vi "DualMotor.vi"() -> ()   [LabVIEW 2020]
uses:
  <vilib>/Platform/TimedLoop/XDataNode/timing_clust.ctl
  <vilib>/Platform/TimedLoop/XDataNode/nitl_modes.ctl
  <vilib>/Platform/TimedLoop/XDataNode/wakeup.ctl
  <vilib>/CANopenLib/CANOPEN.llb/CANopen Interface Create.vi
  <vilib>/CANopenLib/CANOPEN.llb/CANopen SDO Create.vi
  <vilib>/CANopenLib/CANOPEN.llb/CANopen SDO Write [I16].vi
  <vilib>/CANopenLib/CANOPEN.llb/CANopen SDO Close.vi
  <vilib>/CANopenLib/CANOPEN.llb/CANopen SYNC Create.vi
  <vilib>/CANopenLib/CANOPEN.llb/CANopen RPDO Create.vi
  <vilib>/CANopenLib/CANOPEN.llb/CANopen TPDO Create.vi
  <vilib>/CANopenLib/CANOPEN.llb/CANopen TPDO Start.vi
  <vilib>/CANopenLib/CANOPEN.llb/CANopen SYNC Start.vi
  <vilib>/CANopenLib/CANOPEN.llb/CANopen RPDO Start.vi
  <vilib>/imath/engines/lvmath/Functions/Error Handling/MergeErrorsWrapper.vi
  <vilib>/imath/engines/lvmath2/RunTimeEngine/NodeEndStatement/NIMS_NodeEndStatement_Output.vi
  <instcachedir>/0/NIMS_NodeEndStatement_Output_53EC0D466D134D7ABD903AC30B43404B.lvgen/NIMS_NodeEndStatement_Output_53EC0D466D134D7ABD903AC30B43404B_010.vi
  <vilib>/imath/engines/lvmath2/RunTimeEngine/ErrorHandling/NIMS_Finalize Error.vi
  <instcachedir>/0/NIMS_NodeEndStatement_Output_53EC0D466D134D7ABD903AC30B43404B.lvgen/NIMS_NodeEndStatement_Output_53EC0D466D134D7ABD903AC30B43404B_001.vi
  <vilib>/CANopenLib/CANOPEN.llb/CANopen Convert To Data [I16].vi
  <vilib>/CANopenLib/CANOPEN.llb/CANopen Fetch from Data [I16].vi
  <vilib>/CANopenLib/CANOPEN.llb/CANopen Fetch from Data [I32].vi
  <vilib>/CANopenLib/CANOPEN.llb/CANopen SYNC Close.vi
  <vilib>/CANopenLib/CANOPEN.llb/CANopen RPDO Close.vi
  <vilib>/CANopenLib/CANOPEN.llb/CANopen TPDO Close.vi
  <vilib>/CANopenLib/CANOPEN.llb/CANopen Interface Close.vi
  <vilib>/imath/engines/lvmath2/RunTimeEngine/BuiltInFunctions/mod/NIMS_mod_no_size_check.vi
  <instcachedir>/0/NIMS_mod_no_size_check_5393E3382FD241D281EEB71DA286C65B.lvgen/NIMS_mod_no_size_check_5393E3382FD241D281EEB71DA286C65B_001.vi
  <vilib>/FPGAPlugInAG/cRIO-9047/niLvFpga_Open_cRIO-9047.vi
  <vilib>/rvi/interface/common/dynamic/niFpgaDynamicAddResources.vi
  <vilib>/FPGAPlugInAG/Dynamic/niLvFpga_Download_Dynamic.vi
  <vilib>/FPGAPlugInAG/Dynamic/niLvFpga_Reset_Dynamic.vi
  <vilib>/FPGAPlugInAG/Dynamic/niLvFpga_Run_Dynamic.vi
  <vilib>/Utility/error.llb/Error Cluster From Error Code.vi
  <vilib>/rvi/errors/niLvFpgaAdjustHostInterfaceError.vi
  <vilib>/FPGAPlugInAG/Dynamic/niLvFpga_Close_Dynamic.vi
  <vilib>/Platform/TimedLoop/XDataNode/XDataNode.xnode
  <vilib>/rvi/interface/nirviOpenFPGA/nirviOpenFPGA.xnode
  PressureIO_12.vi
  <vilib>/rvi/interface/nirviMethod/nirviMethod.xnode
  <vilib>/rvi/interface/nirviReadWriteControl/nirviReadWriteControl.xnode
  <vilib>/rvi/interface/nirviCloseFPGA/nirviCloseFPGA.xnode
  <vilib>/Platform/TimedLoop/XDataNode/XDNodeRunTimeDep.lvlib
  NiFpgaLv.dll
  <vilib>/rvi/interface/Simulation/niFpgaSimulationCallBeginRW.vi
panel:
  out "L":dbl(graph)
  out "P2":dbl(graph)
  out "P1":dbl(graph)
  out "P2":dbl
  out "P1":dbl
  out "t":dbl
  out "Theta":dbl(graph)
  in  "自定义速度2":dbl
  in  "手动输入速度2":bool
  in  "自定义速度1":dbl
  in  "手动输入速度1":bool
  in  "SaveData?":bool=TRUE
  in  "文件路径（使用对话框）":path=path "C:/data.bin"
  in  "node-ID  2":u8=2 min=1 max=127 step=1
  out "completion code 5":u32
  in  "buffer size (0) 4":u16
  in  "TPDO channel 2":u8(ring)=2 items=["PDO 1", "PDO 2", "PDO 3", "PDO 4"]
  in  "Set Target Vilocity 2":i16
  in  "stop 2":bool
  out "timestamp 2":timestamp=timestamp(3824613290.037175 s since 1904-01-01)
  out "电机绝对位置 2":i32=443333152
  out "速度反馈值 2":i32=300
  in  "目标速度  2":i16
  out "转矩反馈值 0.1% 2":i16=40
  in  "buffer size (0) 3":u16=10
  in  "TPDO channel read 2":u8(ring)=1 items=["PDO 1", "PDO 2", "PDO 3", "PDO 4"]
  in  "RPDO channel write 2":u8(ring)=1 items=["PDO 1", "PDO 2", "PDO 3", "PDO 4"]
  in  "period (ms) 2":i64=10
  out "completion code 4":u32
  out "completion code 3":u32
  in  "batch SDO name 2":string="NiMotion_VM"
  out "completion code":u32
  in  "buffer size (0) 2":u16
  in  "TPDO channel":u8(ring)=2 items=["PDO 1", "PDO 2", "PDO 3", "PDO 4"]
  in  "Set Target Vilocity":i16
  in  "stop":bool
  out "timestamp":timestamp=timestamp(3833513217.6669617 s since 1904-01-01)
  out "电机绝对位置":i32=147770
  out "速度反馈值":i32
  in  "目标速度":i16
  out "转矩反馈值 0.1%":i16=10
  in  "buffer size (0)":u16=10
  in  "TPDO channel read":u8(ring)=1 items=["PDO 1", "PDO 2", "PDO 3", "PDO 4"]
  in  "RPDO channel write":u8(ring)=1 items=["PDO 1", "PDO 2", "PDO 3", "PDO 4"]
  in  "period (ms)":i64=10
  out "completion code 2":u32
  out "completion code 1":u32
  in  "batch SDO name":string="NiMotion_VM"
  in  "node-ID":u8=1 min=1 max=127 step=1
  in  "baud rate":u32(ring) items=["1 Mbit/s"=0, "800 kbit/s"=1, "500 kbit/s"=2, "250 kbit/s"=3, "125 kbit/s"=4, "50 kbit/s"=6, "20 kbit/s"=7, "10 kbit/s"=8]
  in  "CANopen interface":u32(ring) items=["CANopen01", "CANopen02", "CANopen03", "CANopen04", "CANopen05", "CANopen06", "CANopen07", "CANopen08", "CANopen09", "CANopen10", "CANopen11", "CANopen12", "CANopen13", "CANopen14", "CANopen15", "CANopen16", "CANopen17", "CANopen18", "CANopen19", "CANopen20", "CANopen21", "CANopen22", "CANopen23", "CANopen24", "CANopen25", "CANopen26", "CANopen27", "CANopen28", "CANopen29", "CANopen30", "CANopen31", "CANopen32"]
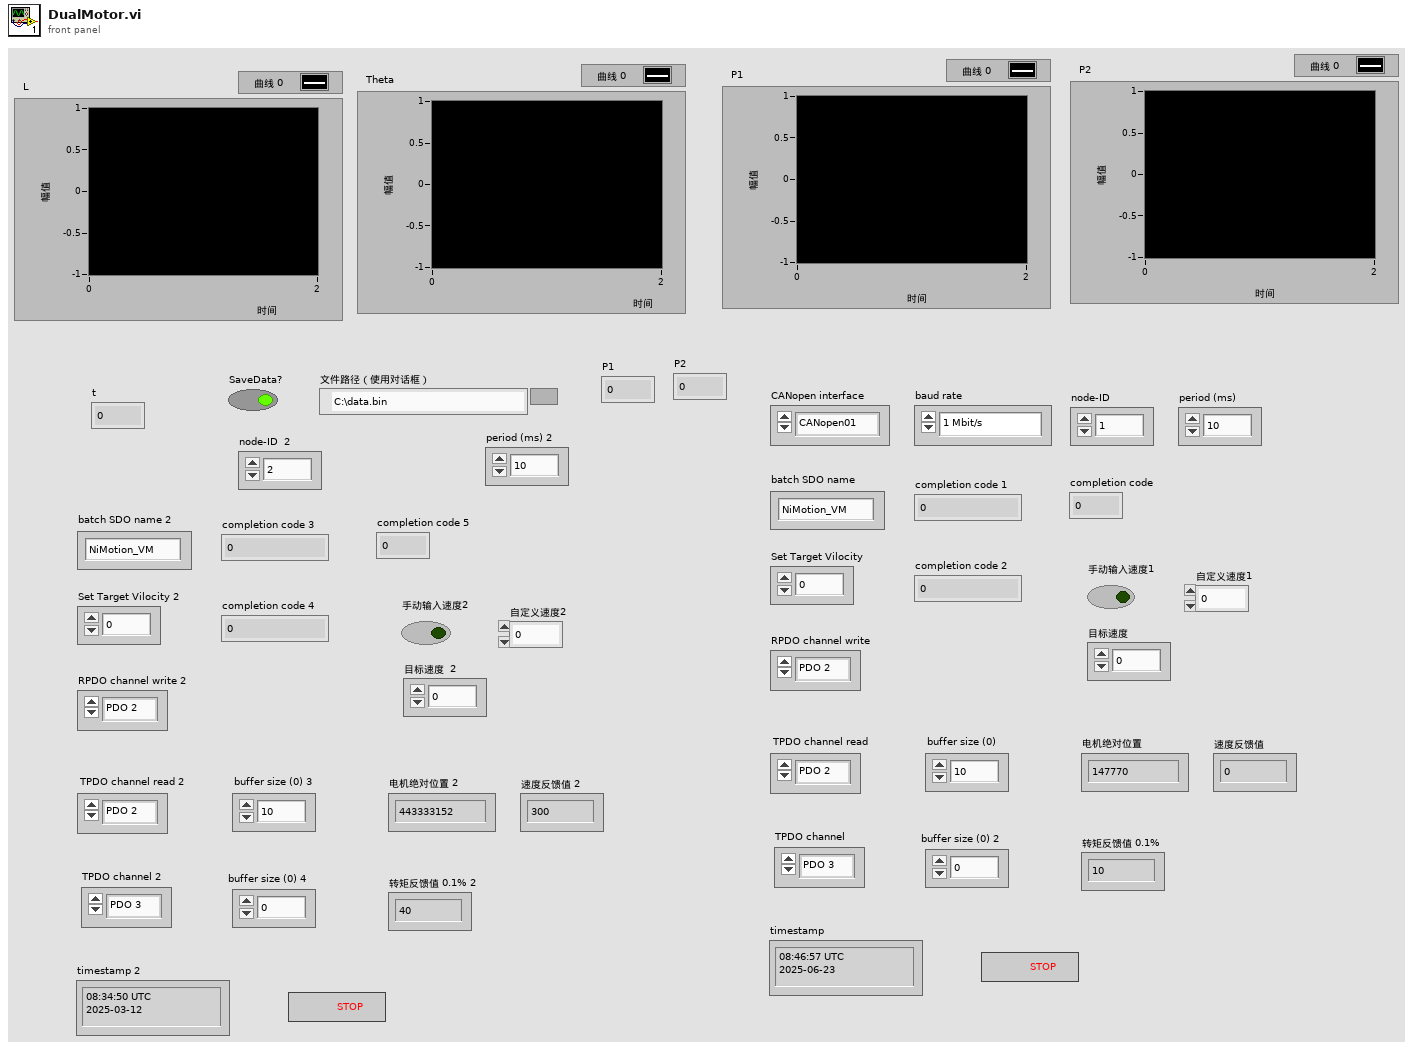
[diagram p1: front panel]
types:
  T1 = enum16{"open", "replace", "create", "open or create", "replace or create", "replace or create with confirmation"}
  T2 = enum16{"big-endian, network order", "native, host order", "little-endian"}
  T3 = typedef "XDNodeRunTimeDep.lvlib/timing_clust.ctl" = cluster{"Expected End [f-1]":u64, "Actual End [f-1]":u64, "Finished Late? [f-1]":bool, "Expected End [i-1]":u64, "Actual End [i-1]":u64, "Finished Late? [i-1]":bool, "Expected Start [i]":u64, "Actual Start [i]":u64, "Expected Start [f]":u64, "Actual Start [f]":u64, "Source Name":string, "Structure Name":string, "Period":i64, "Deadline":i64, "Offset":i64, "Start":i64, "Priority":i32, "Timeout":i32, "Mode":T4, "Wakeup Reason":T5, "Error":errorcluster, "Source Type":string, "Secondary Source Type":string, "Global End Time":u64, "Global Start Time":u64, "Frame Duration":u64, "Iteration Duration":u64, "Assigned CPU":i32, "I/O Scan Engine Mode":u32}
  T4 = typedef "XDNodeRunTimeDep.lvlib/nitl_modes.ctl" = enum32{"No Change", "Process missed periods, maintain original phase", "Discard missed periods, maintain original phase", "Process missed periods, ignore original phase", "Discard missed periods, ignore original phase"}
  T5 = typedef "XDNodeRunTimeDep.lvlib/wakeup.ctl" = enum32{"Normal", "Aborted", "Asynchronous wakeup", "Timing source error", "Timed loop error", "Timeout"}
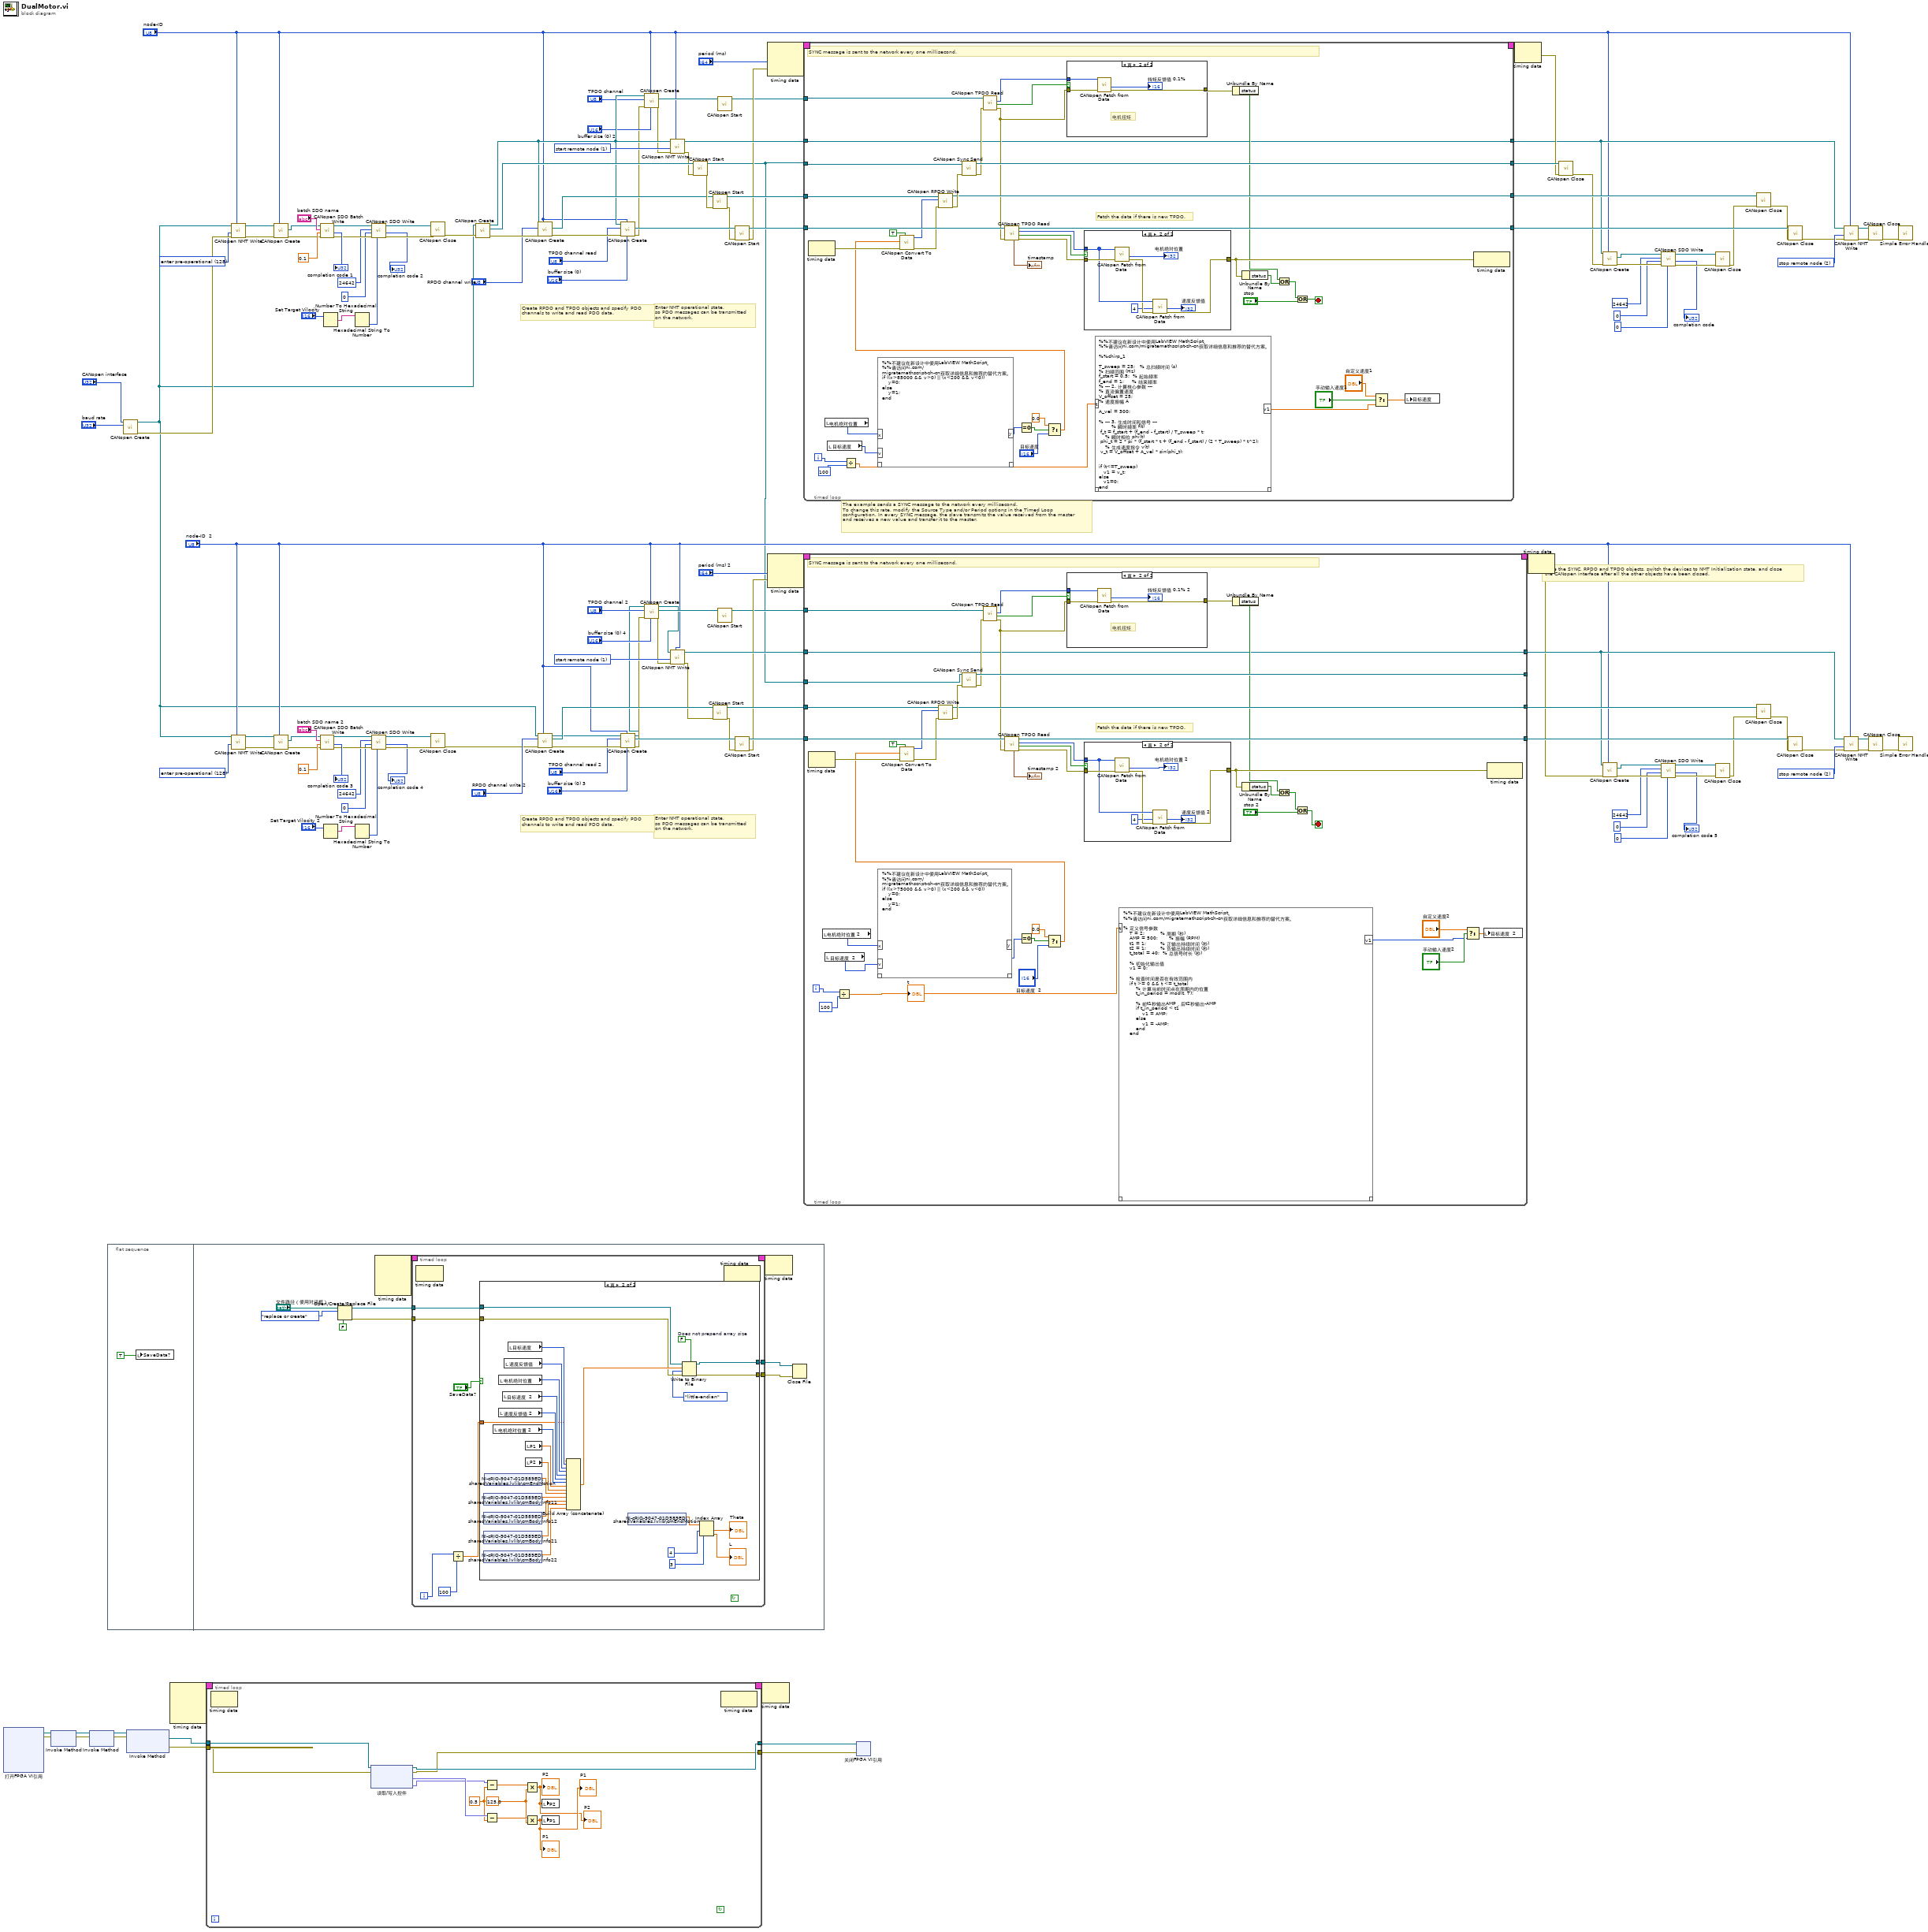
[diagram p0: block diagram]
diagram:
  w52 = u16 2 items=["start remote node"=1, "stop remote node"=2, "enter pre-operational"=128, "reset node"=129, "reset communication"=130] ("command")
  w60 = u16 1 items=["start remote node"=1, "stop remote node"=2, "enter pre-operational"=128, "reset node"=129, "reset communication"=130] ("command")
  w74 = u16 128 items=["start remote node"=1, "stop remote node"=2, "enter pre-operational"=128, "reset node"=129, "reset communication"=130] ("command")
  w112 = u16 2 items=["start remote node"=1, "stop remote node"=2, "enter pre-operational"=128, "reset node"=129, "reset communication"=130] ("command")
  w123 = u16 1 items=["start remote node"=1, "stop remote node"=2, "enter pre-operational"=128, "reset node"=129, "reset communication"=130] ("command")
  w139 = u16 128 items=["start remote node"=1, "stop remote node"=2, "enter pre-operational"=128, "reset node"=129, "reset communication"=130] ("command")
  # "SYNC message is sent to the network every one millisecond."
  # "Enter NMT operational state,\nso PDO messages can be transmitted\non the network."
  # "Create RPDO and TPDO objects and specify PDO \nchannels to write and read PDO data."
  # "SYNC message is sent to the network every one millisecond."
  # "Close the SYNC, RPDO and TPDO objects, switch the devices to NMT Initialization state, and close\n the CANopen interface after all the other objects have been closed."
  # "The example sends a SYNC message to the network every millisecond.\nTo change this rate, modify the Source Type and/or Period options in the Timed Loop\nconfiguration. In every SYNC message, the slave transmits the value received from the master\nand receives a new value and transfer it to the master."
  # "Enter NMT operational state,\nso PDO messages can be transmitted\non the network."
  # "Create RPDO and TPDO objects and specify PDO \nchannels to write and read PDO data."
  n1 = xnode "打开FPGA VI引用"() -> ("FPGA VI引用输出"=w10:refnum<k20>, "错误输出"=w5:errorcluster)  [unwired: 2 in]
  n2 = xnode "Invoke Method"("FPGA VI引用输入"=w10, "错误输入"=w5) -> ("FPGA VI引用输出"=w9:refnum<k20>, "错误输出"=w4:errorcluster)
  n3 = xnode "Invoke Method"("FPGA VI引用输入"=w9, "错误输入"=w4) -> ("FPGA VI引用输出"=w8:refnum<k20>, "错误输出"=w3:errorcluster)
  n4 = flat-sequence {
    frame #0 {
      n5 = local write "SaveData?"(TRUE ("SaveData?")) -> ()
    }
    frame #1 {
      n6 = Open/Create/Replace File(file path (use dialog)="文件路径（使用对话框）", operation (0:open)=T1."replace or create", disable buffering (F)=FALSE ("禁用缓存(F)")) -> (refnum out=w155:refnum<file>, error out=w153:errorcluster)  [unwired: 3 in, 1 out]
      n7 = node-c288() -> (w158:T3)  [unwired: 4 in]
      n8 = timed-loop {
        timing: w158 -> [_]
        timing-out: [_] -> w157
        tunnel: w155 -> [w166]
        tunnel: [w165] -> w154
        tunnel: w153 -> [w164]
        tunnel: [w163] -> w152
        i -> [w161]
        stop <- _ continue-if-true
        n9 = node-c288() -> ()  [unwired: 1 in, 1 out]
        n10 = Divide(x=w161, y=100) -> (x/y=w159:dbl)
        n11 = case shown="真" "SaveData?" {
          tunnel: w166 -> [w168 w193]
          tunnel: [w168 w192] -> w165
          tunnel: w164 -> [w167 w191]
          tunnel: [w167 w190] -> w163
          tunnel: w159 -> [_ w176]
          frame False {
          }
          frame True {
            w189 = FALSE  # Does not prepend array size
            n12 = shared-variable "NI-cRIO-9047-01D589ED\\sharedVariables.lvlib\\cmBodyInfo11"() -> (w180:dbl[])  [unwired: 1 in, 1 out]
            n13 = shared-variable "NI-cRIO-9047-01D589ED\\sharedVariables.lvlib\\cmBodyInfo12"() -> (w179:dbl[])  [unwired: 1 in, 1 out]
            n14 = shared-variable "NI-cRIO-9047-01D589ED\\sharedVariables.lvlib\\cmBodyInfo21"() -> (w178:dbl[])  [unwired: 1 in, 1 out]
            n15 = shared-variable "NI-cRIO-9047-01D589ED\\sharedVariables.lvlib\\cmBodyInfo22"() -> (w177:dbl[])  [unwired: 1 in, 1 out]
            n16 = shared-variable "NI-cRIO-9047-01D589ED\\sharedVariables.lvlib\\cmEndMotion"() -> (w181:dbl[])  [unwired: 1 in, 1 out]
            n17 = local read "电机绝对位置 2"() -> (w182:i32)
            n18 = local read "电机绝对位置"() -> (w185:i32)
            n19 = local read "速度反馈值 2"() -> (w183:i32)
            n20 = local read "目标速度  2"() -> (w184:i16)
            n21 = local read "速度反馈值"() -> (w186:i32)
            n22 = local read "目标速度"() -> (w187:i16)
            n23 = local read "P1"() -> (w172:dbl)
            n24 = local read "P2"() -> (w171:dbl)
            n25 = Build Array (concatenate)(w176, w187, w186, w185, w184, w183, w182, w172, w171, w181, w180, w179, w178, w177) -> (w194:dbl[])
            n26 = shared-variable "NI-cRIO-9047-01D589ED\\sharedVariables.lvlib\\cmEndMotion"() -> (w175:dbl[])  [unwired: 1 in, 1 out]
            n27 = Write to Binary File(file (use dialog)=w193, data=w194, error in=w191, 5:w189, 9:T2."little-endian" ("字节顺序(0:big-endian, network order)")) -> (refnum out=w192:refnum<file>, error out=w190:errorcluster)  [unwired: 1 in, 1 out]
            n28 = Index Array(array=w175, index #1=4, index #2=3) -> (element #1=→"Theta":dbl, element #2=→"L":dbl)
          }
        }
        n29 = node-c288() -> ()  [unwired: 1 in, 1 out]
      }
      n30 = node-c288(w157) -> ()  [unwired: 1 out]
      n31 = Close File(refnum=w154, error in=w152) -> ()  [unwired: 2 out]
    }
  }
  n32 = call-poly <vilib>:"CANopen Create.vi"("baud rate"="baud rate", "interface name"="CANopen interface") -> ("error out"=w140:errorcluster, "interface object out"=w19:refnum<k20>)  [unwired: 8 in]
  n33 = xnode "Invoke Method"("FPGA VI引用输入"=w8, "错误输入"=w3) -> ("FPGA VI引用输出"=w7:refnum<k20>, "错误输出"=w2:errorcluster)  [unwired: 1 in]
  n34 = node-c288() -> (w12:T3)  [unwired: 4 in]
  n35 = timed-loop {
    timing: w12 -> [_]
    timing-out: [_] -> w11
    tunnel: w7 -> [w210]
    tunnel: [w209] -> w6
    tunnel: w2 -> [w208]
    tunnel: [w207] -> w1
    stop <- _ continue-if-true
    w201 = 125.0
    w203 = 0.5
    n36 = node-c288() -> ()  [unwired: 1 in, 1 out]
    n37 = xnode "读取/写入控件"("FPGA VI引用输入"=w210, "错误输入"=w208) -> ("FPGA VI引用输出"=w209:refnum<k20>, "错误输出"=w207:errorcluster, "Chamber_P1"=w206:fxp<+/-,24,5>, "Chamber_P2"=w204:fxp<+/-,24,5>)
    n38 = Subtract(x=w204, y=w203) -> (x-y=w202:dbl)
    n39 = Subtract(x=w206, y=w203) -> (x-y=w205:dbl)
    n40 = Multiply(x=w202, y=w201) -> (x*y=w199:dbl)
    "P2" <- w199
    "P2" <- w199
    n41 = Multiply(x=w205, y=w201) -> (x*y=w200:dbl)
    "P1" <- w200
    "P1" <- w200
    n42 = local write "P2"(w199) -> ()
    n43 = local write "P1"(w200) -> ()
    n44 = node-c288() -> ()  [unwired: 1 in, 1 out]
  }
  n45 = call <vilib>:"CANopen NMT Write.vi"("node-ID (0)"="node-ID", "error in (no error)"=w140, "command"=w139, "interface object in"=w19) -> ("error out"=w143:errorcluster, "interface object out"=w144:refnum<k20>)  [unwired: 6 in]
  n46 = call <vilib>:"CANopen NMT Write.vi"("node-ID (0)"="node-ID  2", "command"=w74, "interface object in"=w19) -> ("error out"=w75:errorcluster, "interface object out"=w76:refnum<k20>)  [unwired: 7 in]
  n47 = call-poly <vilib>:"CANopen Create.vi"("node-ID"="node-ID", "error in (no error)"=w143, "interface object in"=w144) -> ("error out"=w130:errorcluster, "SDO object out"=w136:refnum<k20>)  [unwired: 6 in, 1 out]
  n48 = call-poly <vilib>:"CANopen Create.vi"("node-ID"="node-ID  2", "error in (no error)"=w75, "interface object in"=w76) -> ("error out"=w65:errorcluster, "SDO object out"=w71:refnum<k20>)  [unwired: 6 in, 1 out]
  n49 = call <vilib>:"CANopen SDO Batch Write.vi"("error in (no error)"=w130, "timeout (1s)"=0.1 ("timeout (0s)"), "batch SDO name"="batch SDO name", "SDO object in"=w136) -> ("error out"=w131:errorcluster, "completion code"=→"completion code 1":u32, "SDO object out"=w134:refnum<k20>)  [unwired: 5 in]
  n50 = call <vilib>:"CANopen SDO Batch Write.vi"("error in (no error)"=w65, "timeout (1s)"=0.1 ("timeout (0s)"), "batch SDO name"="batch SDO name 2", "SDO object in"=w71) -> ("error out"=w66:errorcluster, "completion code"=→"completion code 3":u32, "SDO object out"=w69:refnum<k20>)  [unwired: 5 in]
  n51 = Number To Hexadecimal String(2:"Set Target Vilocity") -> (0:w100:string)  [unwired: 1 in]
  n52 = Number To Hexadecimal String(2:"Set Target Vilocity 2") -> (0:w42:string)  [unwired: 1 in]
  n53 = Hexadecimal String To Number(string=w100) -> (number=w98:u32)  [unwired: 2 in, 1 out]
  n54 = Hexadecimal String To Number(string=w42) -> (number=w40:u32)  [unwired: 2 in, 1 out]
  n55 = call-poly <vilib>:"CANopen SDO Write.vi"("I16 data"=w98, "error in (no error)"=w131, "object sub-index (0)"=u8 0, "object index"=u16 24642, "SDO object in"=w134) -> ("error out"=w132:errorcluster, "completion code"=→"completion code 2":u32, "SDO object out"=w133:refnum<k20>)  [unwired: 4 in]
  n56 = call-poly <vilib>:"CANopen SDO Write.vi"("I16 data"=w40, "error in (no error)"=w66, "object sub-index (0)"=u8 0, "object index"=u16 24642, "SDO object in"=w69) -> ("error out"=w67:errorcluster, "completion code"=→"completion code 4":u32, "SDO object out"=w68:refnum<k20>)  [unwired: 4 in]
  n57 = call-poly <vilib>:"CANopen Close.vi"("error in (no error)"=w132, "SDO object in"=w133) -> ("error out"=w115:errorcluster)  [unwired: 9 in]
  n58 = call-poly <vilib>:"CANopen Close.vi"("error in (no error)"=w67, "SDO object in"=w68) -> ("error out"=w20:errorcluster)  [unwired: 9 in]
  n59 = call-poly <vilib>:"CANopen Create.vi"("error in (no error)"=w115, "interface object in"=w19) -> ("error out"=w125:errorcluster, "SYNC object out"=w124:refnum<k20>, "interface object out"=w96:refnum<k20>)  [unwired: 7 in]
  n60 = call-poly <vilib>:"CANopen Create.vi"("node-ID"="node-ID", "error in (no error)"=w125, "PDO channel"="RPDO channel write", "interface object in"=w96) -> ("error out"=w119:errorcluster, "RPDO object out"=w118:refnum<k20>)  [unwired: 5 in, 1 out]
  n61 = call-poly <vilib>:"CANopen Create.vi"("node-ID"="node-ID  2", "error in (no error)"=w20, "PDO channel"="RPDO channel write 2", "interface object in"=w19) -> ("error out"=w58:errorcluster, "RPDO object out"=w57:refnum<k20>, "interface object out"=w18:refnum<k20>)  [unwired: 5 in]
  n62 = call-poly <vilib>:"CANopen Create.vi"("buffer size (0)"="buffer size (0)", "node-ID"="node-ID", "error in (no error)"=w119, "PDO channel"="TPDO channel read", "interface object in"=w96) -> ("error out"=w91:errorcluster, "TPDO object out"=w127:refnum<k20>)  [unwired: 4 in, 1 out]
  n63 = call-poly <vilib>:"CANopen Create.vi"("buffer size (0)"="buffer size (0) 3", "node-ID"="node-ID  2", "error in (no error)"=w58, "PDO channel"="TPDO channel read 2", "interface object in"=w18) -> ("error out"=w34:errorcluster, "TPDO object out"=w62:refnum<k20>, "interface object out"=w17:refnum<k20>)  [unwired: 4 in]
  n64 = call-poly <vilib>:"CANopen Create.vi"("buffer size (0)"="buffer size (0) 2", "node-ID"="node-ID", "error in (no error)"=w91, "PDO channel"="TPDO channel", "interface object in"=w96) -> ("error out"=w90:errorcluster, "TPDO object out"=w93:refnum<k20>)  [unwired: 4 in, 1 out]
  n65 = call-poly <vilib>:"CANopen Create.vi"("buffer size (0)"="buffer size (0) 4", "node-ID"="node-ID  2", "error in (no error)"=w34, "PDO channel"="TPDO channel 2", "interface object in"=w17) -> ("error out"=w33:errorcluster, "TPDO object out"=w36:refnum<k20>, "interface object out"=w16:refnum<k20>)  [unwired: 4 in]
  n66 = call <vilib>:"CANopen NMT Write.vi"("node-ID (0)"="node-ID", "error in (no error)"=w90, "command"=w123, "interface object in"=w96) -> ("error out"=w122:errorcluster, "interface object out"=w104:refnum<k20>)  [unwired: 6 in]
  n67 = call <vilib>:"CANopen NMT Write.vi"("node-ID (0)"="node-ID  2", "error in (no error)"=w33, "command"=w60, "interface object in"=w16) -> ("error out"=w15:errorcluster, "interface object out"=w46:refnum<k20>)  [unwired: 6 in]
  n68 = call-poly <vilib>:"CANopen Start.vi"("error in (no error)"=w122, "SYNC object in"=w124) -> ("error out"=w121:errorcluster, "SYNC object out"=w14:refnum<k20>)  [unwired: 8 in]
  n69 = call-poly <vilib>:"CANopen Start.vi"("error in (no error)"=w121, "RPDO object in"=w118) -> ("error out"=w120:errorcluster, "RPDO object out"=w103:refnum<k20>)  [unwired: 8 in]
  n70 = call-poly <vilib>:"CANopen Start.vi"("error in (no error)"=w15, "RPDO object in"=w57) -> ("error out"=w59:errorcluster, "RPDO object out"=w45:refnum<k20>)  [unwired: 8 in]
  n71 = call-poly <vilib>:"CANopen Start.vi"("TPDO object in"=w93) -> ("TPDO object out"=w92:refnum<k20>)  [unwired: 9 in, 1 out]
  n72 = call-poly <vilib>:"CANopen Start.vi"("TPDO object in"=w36) -> ("TPDO object out"=w35:refnum<k20>)  [unwired: 9 in, 1 out]
  n73 = call-poly <vilib>:"CANopen Start.vi"("error in (no error)"=w120, "TPDO object in"=w127) -> ("error out"=w101:errorcluster, "TPDO object out"=w102:refnum<k20>)  [unwired: 8 in]
  n74 = call-poly <vilib>:"CANopen Start.vi"("error in (no error)"=w59, "TPDO object in"=w62) -> ("error out"=w43:errorcluster, "TPDO object out"=w44:refnum<k20>)  [unwired: 8 in]
  n75 = node-c288(w11) -> ()  [unwired: 1 out]
  n76 = node-c288("period (ms)", w101) -> (w148:T3)  [unwired: 1 in]
  n77 = node-c288("period (ms) 2", w43) -> (w146:T3)  [unwired: 1 in]
  n78 = timed-loop {
    timing: w148 -> [_]
    timing-out: [_] -> w147
    tunnel: w14 -> [w254]
    tunnel: [w244] -> w108
    tunnel: [w227] -> w88
    tunnel: w104 -> [w227]
    tunnel: w103 -> [w248]
    tunnel: w102 -> [w249]
    tunnel: [w246] -> w111
    tunnel: [w245] -> w89
    tunnel: w92 -> [w237]
    i -> [w219]
    stop <- w253 stop-if-true
    # "Fetch the data if there is new TPDO."
    n79 = node-c288() -> (w239:errorcluster)  [unwired: 1 in]
    n80 = local read "电机绝对位置"() -> (w226:i32)
    n81 = local read "目标速度"() -> (w220:i16)
    n82 = Divide(x=w219, y=100) -> (x/y=w217:dbl)
    n83 = mathscript code="%%不建议在新设计中使用LabVIEW MathScript。\n%%请访问ni.com/migratemathscript-zh-cn获取详细信息和推荐的替代方案。\nif ((x>85000 && v>0) || (x<200 && v<0))\n    y=0;\nelse\n    y=1;\nend"("x"=w226, "v"=w220) -> ("y"=w225:i32)  [unwired: 1 in, 1 out]
    n84 = Equal To 0?(x=w225) -> (x = 0?=w224:bool)
    n85 = Select(t=0.0, s=w224, f="目标速度") -> (s? t:f=w221:dbl)
    n86 = call-poly <vilib>:"CANopen Convert To Data.vi"("trim"=TRUE, "error in (no error)"=w239, "signed 16-bit integer"=w221) -> ("error out"=w228:errorcluster, "CANopen data out"=w238:u8[])  [unwired: 7 in]
    n87 = call <vilib>:"CANopen RPDO Write.vi"("error in (no error)"=w228, "data"=w238, "RPDO object in"=w248) -> ("error out"=w247:errorcluster, "RPDO object out"=w245:refnum<k20>)  [unwired: 7 in]
    n88 = call <vilib>:"CANopen Sync Send.vi"("error in (no error)"=w247, "SYNC object in"=w254) -> ("error out"=w236:errorcluster, "SYNC object out"=w244:refnum<k20>)  [unwired: 8 in]
    n89 = call <vilib>:"CANopen TPDO Read.vi"("error in (no error)"=w236, "TPDO object in"=w237) -> ("error out"=w233:errorcluster, "new data?"=w234:bool, "data"=w235:u8[])  [unwired: 5 in, 2 out]
    n90 = call <vilib>:"CANopen TPDO Read.vi"("error in (no error)"=w233, "TPDO object in"=w249) -> ("error out"=w250:errorcluster, "new data?"=w243:bool, "data"=w241:u8[], "TPDO object out"=w246:refnum<k20>, "timestamp"=→"timestamp":timestamp)  [unwired: 5 in]
    n91 = case shown="真" w234 {
      tunnel: w233 -> [w416 w420]
      tunnel: w235 -> [_ w419]
      tunnel: [w416 w418] -> w232
      frame False {
      }
      frame True {
        # "电机扭矩"
        n92 = call-poly <vilib>:"CANopen Fetch from Data.vi"("error in (no error)"=w420, "CANopen data in"=w419) -> ("error out"=w418:errorcluster, "signed 16-bit integer"=→"转矩反馈值 0.1%":i16)  [unwired: 7 in, 1 out]
      }
    }
    n93 = case shown="真" w243 {
      tunnel: w250 -> [w426 w433]
      tunnel: w241 -> [_ w432]
      tunnel: [w426 w430] -> w242
      frame False {
      }
      frame True {
        n94 = call-poly <vilib>:"CANopen Fetch from Data.vi"("error in (no error)"=w433, "CANopen data in"=w432) -> ("error out"=w431:errorcluster, "signed 32-bit integer"=→"电机绝对位置":i32)  [unwired: 7 in, 1 out]
        n95 = call-poly <vilib>:"CANopen Fetch from Data.vi"("error in (no error)"=w431, "offset (0)"=u32 4, "CANopen data in"=w432) -> ("error out"=w430:errorcluster, "signed 32-bit integer"=→"速度反馈值":i32)  [unwired: 6 in, 1 out]
      }
    }
    n96 = mathscript code="%%不建议在新设计中使用LabVIEW MathScript。\n%%请访问ni.com/migratemathscript-zh-cn获取详细信息和推荐的替代方案。\n\n%%chirp_1\n\nT_sweep = 25;   % 总扫频时间 (s)\n% 扫频范围 (Hz)\nf_start = 0.5;  % 起始频率\nf_end = 1;     % 结束频率\n% --- 2. 计算核心参数 ---\n% 直流偏置速度\nV_offset = 25;\n% 速度振幅 A\n\nA_vel = 300;\n\n% --- 3. 生成时间和信号 ---\n        % 瞬时频率 f(t)\n f_t = f_start + (f_end - f_start) / T_sweep * t;\n    % 瞬时相位 phi(t)\n phi_t = 2 * pi * (f_start * t + (f_end - f_start) / (2 * T_sweep) * t^2);\n    % 生成速度指令 v(t)\n v_t = V_offset + A_vel * sin(phi_t);\n\n\nif (t<=T_sweep)\n   v1 = v_t;\nelse\n   v1=0;\nend"("t"=w217) -> ("v1"=w215:dbl)  [unwired: 1 in, 1 out]
    n97 = Unbundle By Name(w232) -> ("status"=w230:bool)
    n98 = Unbundle By Name(w242) -> ("status"=w231:bool)
    n99 = Or(x=w230, y=w231) -> (x .or. y?=w229:bool)
    n100 = Or(x=w229, y="stop") -> (x .or. y?=w253:bool)
    n101 = Select(t="自定义速度1", s="手动输入速度1", f=w215) -> (s? t:f=w213:dbl)
    n102 = local write "目标速度"(w213) -> ()
    n103 = node-c288(w242) -> ()  [unwired: 1 out]
  }
  n104 = timed-loop {
    timing: w146 -> [_]
    timing-out: [_] -> w145
    tunnel: [w466] -> _
    tunnel: [w449] -> w31
    tunnel: w46 -> [w449]
    tunnel: w45 -> [w470]
    tunnel: w44 -> [w471]
    tunnel: [w468] -> w51
    tunnel: [w467] -> w32
    tunnel: w35 -> [w459]
    tunnel: w14 -> [w441]
    i -> [w438]
    stop <- w475 stop-if-true
    # "Fetch the data if there is new TPDO."
    n105 = node-c288() -> (w461:errorcluster)  [unwired: 1 in]
    n106 = local read "电机绝对位置 2"() -> (w448:i32)
    n107 = local read "目标速度  2"() -> (w442:i16)
    n108 = Divide(x=w438, y=100) -> (x/y=w436:dbl)
    "t" <- w436
    n109 = mathscript code="%%不建议在新设计中使用LabVIEW MathScript。\n%%请访问ni.com/migratemathscript-zh-cn获取详细信息和推荐的替代方案。\nif ((x>75000 && v>0) || (x<200 && v<0))\n    y=0;\nelse\n    y=1;\nend"("x"=w448, "v"=w442) -> ("y"=w447:i32)  [unwired: 1 in, 1 out]
    n110 = Equal To 0?(x=w447) -> (x = 0?=w446:bool)
    n111 = Select(t=0.0, s=w446, f="目标速度  2") -> (s? t:f=w443:dbl)
    n112 = call-poly <vilib>:"CANopen Convert To Data.vi"("trim"=TRUE, "error in (no error)"=w461, "signed 16-bit integer"=w443) -> ("error out"=w450:errorcluster, "CANopen data out"=w460:u8[])  [unwired: 7 in]
    n113 = call <vilib>:"CANopen RPDO Write.vi"("error in (no error)"=w450, "data"=w460, "RPDO object in"=w470) -> ("error out"=w469:errorcluster, "RPDO object out"=w467:refnum<k20>)  [unwired: 7 in]
    n114 = call <vilib>:"CANopen Sync Send.vi"("error in (no error)"=w469, "SYNC object in"=w441) -> ("error out"=w458:errorcluster, "SYNC object out"=w466:refnum<k20>)  [unwired: 8 in]
    n115 = call <vilib>:"CANopen TPDO Read.vi"("error in (no error)"=w458, "TPDO object in"=w459) -> ("error out"=w455:errorcluster, "new data?"=w456:bool, "data"=w457:u8[])  [unwired: 5 in, 2 out]
    n116 = call <vilib>:"CANopen TPDO Read.vi"("error in (no error)"=w455, "TPDO object in"=w471) -> ("error out"=w472:errorcluster, "new data?"=w465:bool, "data"=w463:u8[], "TPDO object out"=w468:refnum<k20>, "timestamp"=→"timestamp 2":timestamp)  [unwired: 5 in]
    n117 = case shown="真" w456 {
      tunnel: w455 -> [w636 w640]
      tunnel: w457 -> [_ w639]
      tunnel: [w636 w638] -> w454
      frame False {
      }
      frame True {
        # "电机扭矩"
        n118 = call-poly <vilib>:"CANopen Fetch from Data.vi"("error in (no error)"=w640, "CANopen data in"=w639) -> ("error out"=w638:errorcluster, "signed 16-bit integer"=→"转矩反馈值 0.1% 2":i16)  [unwired: 7 in, 1 out]
      }
    }
    n119 = case shown="真" w465 {
      tunnel: w472 -> [w646 w653]
      tunnel: w463 -> [_ w652]
      tunnel: [w646 w650] -> w464
      frame False {
      }
      frame True {
        n120 = call-poly <vilib>:"CANopen Fetch from Data.vi"("error in (no error)"=w653, "CANopen data in"=w652) -> ("error out"=w651:errorcluster, "signed 32-bit integer"=→"电机绝对位置 2":i32)  [unwired: 7 in, 1 out]
        n121 = call-poly <vilib>:"CANopen Fetch from Data.vi"("error in (no error)"=w651, "offset (0)"=u32 4, "CANopen data in"=w652) -> ("error out"=w650:errorcluster, "signed 32-bit integer"=→"速度反馈值 2":i32)  [unwired: 6 in, 1 out]
      }
    }
    n122 = mathscript code="%%不建议在新设计中使用LabVIEW MathScript。\n%%请访问ni.com/migratemathscript-zh-cn获取详细信息和推荐的替代方案。\n\n% 定义信号参数\n    T = 2;          % 周期 (秒)\n    AMP = 500;       % 振幅 (RPM)\n    t1 = 1;         % 正输出持续时间 (秒)\n    t2 = 1;         % 负输出持续时间 (秒)\n    t_total = 40;  % 总信号时长 (秒)\n    \n    % 初始化输出值\n    v1 = 0;\n    \n    % 检查时间是否在有效范围内\n    if t >= 0 && t <= t_total\n        % 计算当前时间点在周期内的位置\n        t_in_period = mod(t, T);\n        \n        % 前t1秒输出AMP，后t2秒输出-AMP\n        if t_in_period < t1\n            v1 = AMP;\n        else\n            v1 = -AMP;\n        end\n    end"("t"=w436) -> ("v1"=w434:i32)  [unwired: 1 in, 1 out]
    n123 = Unbundle By Name(w454) -> ("status"=w452:bool)
    n124 = Unbundle By Name(w464) -> ("status"=w453:bool)
    n125 = Or(x=w452, y=w453) -> (x .or. y?=w451:bool)
    n126 = Or(x=w451, y="stop 2") -> (x .or. y?=w475:bool)
    n127 = Select(t="自定义速度2", s="手动输入速度2", f=w434) -> (s? t:f=w435:dbl)
    n128 = local write "目标速度  2"(w435) -> ()
    n129 = node-c288(w464) -> ()  [unwired: 1 out]
  }
  n130 = xnode "关闭FPGA VI引用"("FPGA VI引用输入"=w6, "错误输入"=w1) -> ()  [unwired: 1 out]
  n131 = node-c288(w147) -> (w106:errorcluster)
  n132 = node-c288(w145) -> (w13:errorcluster)
  n133 = call-poly <vilib>:"CANopen Close.vi"("error in (no error)"=w106, "SYNC object in"=w108) -> ("error out"=w85:errorcluster)  [unwired: 9 in]
  n134 = call-poly <vilib>:"CANopen Create.vi"("node-ID"="node-ID", "error in (no error)"=w85, "interface object in"=w88) -> ("error out"=w84:errorcluster, "SDO object out"=w87:refnum<k20>)  [unwired: 6 in, 1 out]
  n135 = call-poly <vilib>:"CANopen Create.vi"("node-ID"="node-ID  2", "error in (no error)"=w13, "interface object in"=w31) -> ("error out"=w28:errorcluster, "SDO object out"=w30:refnum<k20>)  [unwired: 6 in, 1 out]
  n136 = call-poly <vilib>:"CANopen SDO Write.vi"("I16 data"=i16 0, "error in (no error)"=w84, "object sub-index (0)"=u8 0 ("sub-index"), "object index"=u16 24642, "SDO object in"=w87) -> ("error out"=w83:errorcluster, "completion code"=→"completion code":u32, "SDO object out"=w86:refnum<k20>)  [unwired: 4 in]
  n137 = call-poly <vilib>:"CANopen SDO Write.vi"("I16 data"=i16 0, "error in (no error)"=w28, "object sub-index (0)"=u8 0 ("sub-index"), "object index"=u16 24642, "SDO object in"=w30) -> ("error out"=w27:errorcluster, "completion code"=→"completion code 5":u32, "SDO object out"=w29:refnum<k20>)  [unwired: 4 in]
  n138 = call-poly <vilib>:"CANopen Close.vi"("error in (no error)"=w83, "SDO object in"=w86) -> ("error out"=w82:errorcluster)  [unwired: 9 in]
  n139 = call-poly <vilib>:"CANopen Close.vi"("error in (no error)"=w27, "SDO object in"=w29) -> ("error out"=w26:errorcluster)  [unwired: 9 in]
  n140 = call-poly <vilib>:"CANopen Close.vi"("error in (no error)"=w82, "RPDO object in"=w89) -> ("error out"=w110:errorcluster)  [unwired: 9 in]
  n141 = call-poly <vilib>:"CANopen Close.vi"("error in (no error)"=w26, "RPDO object in"=w32) -> ("error out"=w50:errorcluster)  [unwired: 9 in]
  n142 = call-poly <vilib>:"CANopen Close.vi"("error in (no error)"=w110, "TPDO object in"=w111) -> ("error out"=w109:errorcluster)  [unwired: 9 in]
  n143 = call-poly <vilib>:"CANopen Close.vi"("error in (no error)"=w50, "TPDO object in"=w51) -> ("error out"=w49:errorcluster)  [unwired: 9 in]
  n144 = call <vilib>:"CANopen NMT Write.vi"("node-ID (0)"="node-ID", "error in (no error)"=w109, "command"=w112, "interface object in"=w88) -> ("error out"=w114:errorcluster, "interface object out"=w113:refnum<k20>)  [unwired: 6 in]
  n145 = call <vilib>:"CANopen NMT Write.vi"("node-ID (0)"="node-ID  2", "error in (no error)"=w49, "command"=w52, "interface object in"=w31) -> ("error out"=w54:errorcluster, "interface object out"=w53:refnum<k20>)  [unwired: 6 in]
  n146 = call-poly <vilib>:"CANopen Close.vi"("error in (no error)"=w114, "interface object in"=w113) -> ("error out"=w107:errorcluster)  [unwired: 9 in]
  n147 = call-poly <vilib>:"CANopen Close.vi"("error in (no error)"=w54, "interface object in"=w53) -> ("error out"=w48:errorcluster)  [unwired: 9 in]
  n148 = call <vilib>:"Simple Error Handler.vi"("error in (no error)"=w107) -> ()  [unwired: 4 in, 5 out]
  n149 = call <vilib>:"Simple Error Handler.vi"("error in (no error)"=w48) -> ()  [unwired: 4 in, 5 out]
